vi "mHTprofile.vi"(0 "Gamma0":dbl caption="Gamma0 (0)" format="%#_13g", 1 "Gamma2":dbl caption="Gamma2 (0)" format="%#_13g", 2 "Delta0":dbl caption="Delta0 (0)" format="%#_13g", 3 "Delta2":dbl caption="Delta2 (0)" format="%#_13g", 4 "NuOptRe":dbl caption="NuOptRe (0)" format="%#_13g", 5 "NuOptIm":dbl caption="NuOptIm (0)" format="%#_13g", 6 "Xlm":dbl caption="Xlm (0)" format="%#_13g", 7 "nu0":dbl caption="nu0 (0)" format="%#_13g", 8 "Ylm":dbl caption="Ylm (0)" format="%#_13g", 9 "GammaD":dbl caption="GammaD (0)" format="%#_13g", 10 "alpha":dbl=10.0 caption="alpha (10)" format="%#_13g", 11 "nu":dbl format="%#_13g", 12 "disp":enum32{"Absorption", "Dispersion"}(ring) caption="disp (Absorption)") -> (18 "mHT":dbl=nan format="%#_16g")   [LabVIEW 2015]
panel:
  # "modified Hartman Tran profile"
  # "Subroutine to compute the complex normalized spectral-line shape using mHT model\n\nStandard Input Parameters:\n--------------------\nnu0     : Unperturbed line position in cm-1 (default: 0).\nGammaD  : Doppler broadening in cm-1 (default: 0).\nGamma0  : Speed-averaged line-width in cm-1 (default: 0).       \nGamma2  : Quadratic speed dependence parameter of the line-width in cm-1 (default: 0).\nDelta0  : Speed-averaged line-shift in cm-1 (default: 0).\nDelta2  : Quadratic speed dependence parameter of the line-shift in cm-1 (default: 0).   \nNuOptRe : Real part of the complex Dicke parameter in cm-1 (default: 0).\nNuOptIm : Imaginary part of the complex Dicke parameter in cm-1 (default: 0).    \nnu      : Current WaveNumber in cm-1.\nYlm     : Imaginary part of the 1st order (Rosenkranz) line mixing coefficients, dimensionless (default: 0).\nXlm     : Real part of the 1st order (Rosenkranz) line mixing coefficients, dimensionless (default: 0).\nalpha   : Mass ratio in the molecule for calculating beta-correction, applicable up to alpha=5, \n          dimensionless (default: 10).\ndisp    : Boolean trigger for including dispersion profile in the output (default: Absorption).\n\nThe function has one outputs:\n--------------------\n(1)     : Real or imaginary (depending on disp value) part of the normalized spectral shape in cm."
  # "Input Section"
  # "Output Section"
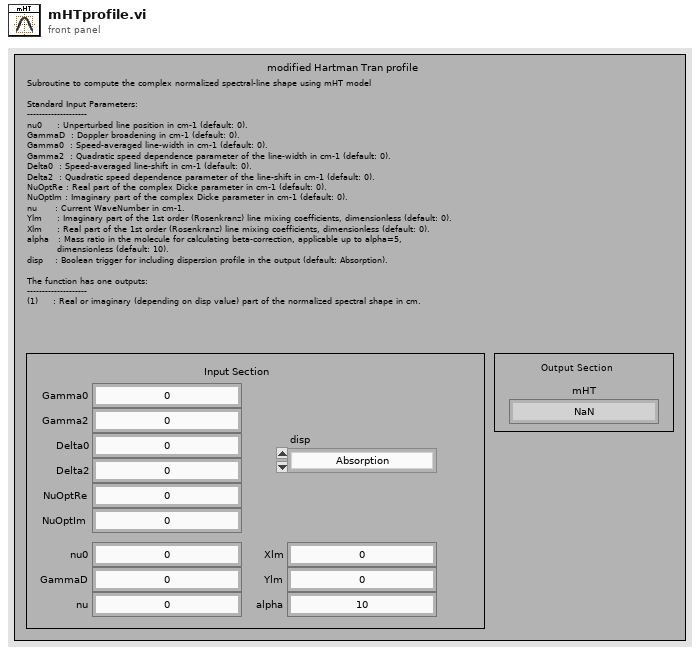
[diagram p1: front panel]
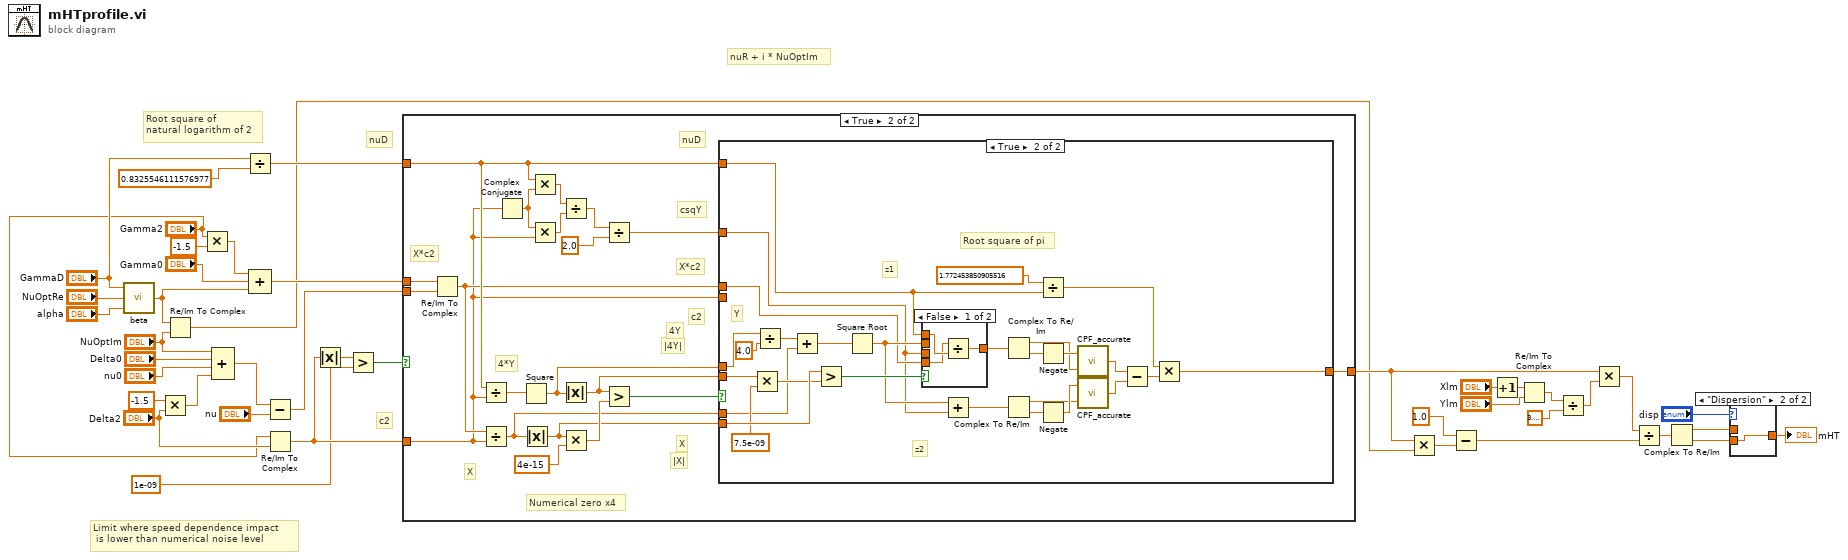
[diagram p0: block diagram]
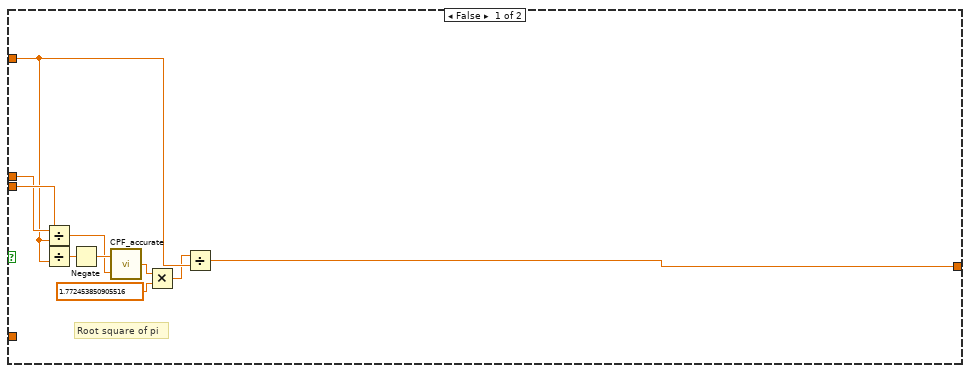
[diagram p3: hidden frame]
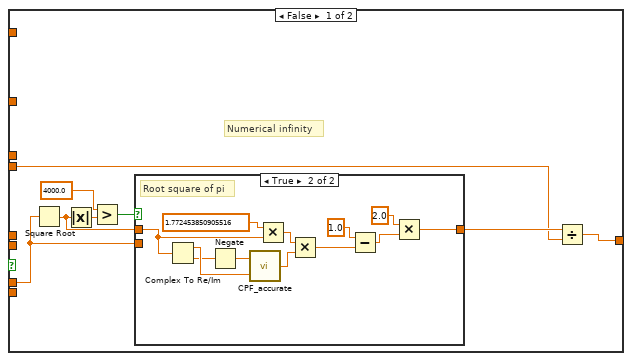
[diagram p4: hidden frame]
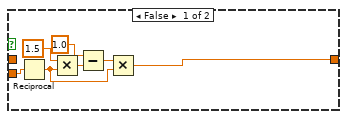
[diagram p5: hidden frame]
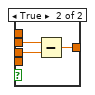
[diagram p6: hidden frame]
diagram:
  # "nuR + i * NuOptIm"
  # "nuD"
  # "c2"
  # "Limit where speed dependence impact\n is lower than numerical noise level"
  # "Root square of\nnatural logarithm of 2"
  n1 = call "beta.vi"("alpha"="alpha", "NuOptRe"="NuOptRe", "GammaD"="GammaD") -> ("nuR"=w11:dbl)
  n2 = Multiply(x=-1.5 ("y"), y="Delta2") -> (x*y=w3:dbl)
  n3 = Re/Im To Complex(1:"NuOptIm", 2:w11) -> (0:w25:cdb)
  n4 = Multiply(x="Gamma2", y=-1.5) -> (x*y=w10:dbl)
  n5 = Compound Arithmetic op=ADD("NuOptIm", "Delta0", "nu0", w3) -> (w2:dbl)
  n6 = Divide(x="GammaD", y=0.8325546111576977 ("sln2")) -> (x/y=w32:dbl)
  n7 = Compound Arithmetic op=ADD(w10, "Gamma0", w11) -> (w34:dbl)
  n8 = Subtract(x=w2, y="nu") -> (x-y=w33:dbl)
  n9 = Re/Im To Complex(1:"Delta2", 2:"Gamma2") -> (0:w6:cdb)
  n10 = Absolute Value(x=w6) -> (abs(x)=w36:dbl)
  n11 = Greater?(x=w36, y=1e-09) -> (0:w35:bool)
  n12 = case shown="True" w35 {
    tunnel: w34 -> [w50 w71]
    tunnel: w33 -> [w51 w55]
    tunnel: w32 -> [w44 w56]
    tunnel: w6 -> [_ w53]
    tunnel: [w42 w57] -> w26
    frame False {
      # "Root square of pi"
      n13 = Divide(x=w50, y=w44) -> (x/y=w47:dbl)
      n14 = Divide(x=w51, y=w44) -> (x/y=w49:dbl)
      n15 = Negate(x=w49) -> (-x=w48:dbl)
      n16 = call "CPF_accurate.vi"("y"=w47, "x"=w48) -> ("CPF Value"=w46:cdb)
      n17 = Multiply(x=w46, y=1.772453850905516) -> (x*y=w43:cdb)
      n18 = Divide(x=w43, y=w44) -> (x/y=w42:cdb)
    }
    frame True {
      # "|4Y|"
      # "4Y"
      # "|X|"
      # "X"
      # "4*Y"
      # "X"
      # "c2"
      # "X*c2"
      # "csqY"
      # "nuD"
      # "X*c2"
      # "Numerical zero x4"
      n19 = Re/Im To Complex(1:w55, 2:w71) -> (0:w54:cdb)
      n20 = Divide(x=w56, y=w53) -> (x/y=w70:cdb)
      n21 = Divide(x=w54, y=w53) -> (x/y=w61:cdb)
      n22 = Complex Conjugate(1:w53) -> (0:w67:cdb)
      n23 = Square(x=w70) -> (x^2=w60:cdb)
      n24 = Absolute Value(x=w61) -> (abs(x)=w59:dbl)
      n25 = Multiply(x=w56, y=w67) -> (x*y=w66:cdb)
      n26 = Multiply(x=w67, y=w53) -> (x*y=w65:cdb)
      n27 = Divide(x=w66, y=w65) -> (x/y=w64:cdb)
      n28 = Absolute Value(x=w60) -> (abs(x)=w58:dbl)
      n29 = Multiply(x=w59, y=4e-15 ("sln2")) -> (x*y=w69:dbl)
      n30 = Divide(x=w64, y=2.0) -> (x/y=w62:cdb)
      n31 = Greater?(x=w58, y=w69) -> (0:w68:bool)
      n32 = case shown="True" w68 {
        tunnel: w62 -> [_ w100]
        tunnel: w61 -> [w76 w114]
        tunnel: w53 -> [w78 _]
        tunnel: w60 -> [_ w123]
        tunnel: w59 -> [_ w118]
        tunnel: w58 -> [_ w117]
        tunnel: w54 -> [_ w101]
        tunnel: w56 -> [_ w99]
        tunnel: [w72 w102] -> w57
        frame False {
          # "Numerical infinity"
          n33 = Square Root(x=w76) -> (sqrt(x)=w73:cdb)
          n34 = Absolute Value(x=w73) -> (abs(x)=w77:dbl)
          n35 = Greater?(x=4000.0 ("sln2"), y=w77) -> (0:w74:bool)
          n36 = case shown="True" w74 {
            tunnel: w76 -> [w86 _]
            tunnel: w73 -> [_ w87]
            tunnel: [w81 w88] -> w79
            frame False {
              n37 = Reciprocal(x=w86) -> (1/x=w80:cdb)
              n38 = Multiply(x=1.5, y=w80) -> (x*y=w84:cdb)
              n39 = Subtract(x=1.0, y=w84) -> (x-y=w82:cdb)
              n40 = Multiply(x=w82, y=w80) -> (x*y=w81:cdb)
            }
            frame True {
              # "Root square of pi"
              n41 = Complex To Re/Im(x + iy=w87) -> (x=w97:dbl, y=w96:dbl)
              n42 = Negate(x=w96) -> (-x=w98:dbl)
              n43 = call "CPF_accurate.vi"("y"=w97, "x"=w98) -> ("CPF Value"=w94:cdb)
              n44 = Multiply(x=1.772453850905516, y=w87) -> (x*y=w93:cdb)
              n45 = Multiply(x=w93, y=w94) -> (x*y=w92:cdb)
              n46 = Subtract(x=1.0, y=w92) -> (x-y=w90:cdb)
              n47 = Multiply(x=2.0, y=w90) -> (x*y=w88:cdb)
            }
          }
          n48 = Divide(x=w79, y=w78) -> (x/y=w72:cdb)
        }
        frame True {
          # "z2"
          # "z1"
          # "Y"
          # "Root square of pi"
          n49 = Multiply(x=w117, y=7.5e-09) -> (x*y=w115:dbl)
          n50 = Divide(x=w123, y=4.0) -> (x/y=w125:cdb)
          n51 = Add(x=w125, y=w114) -> (x+y=w126:cdb)
          n52 = Greater?(x=w118, y=w115) -> (0:w122:bool)
          n53 = Square Root(x=w126) -> (sqrt(x)=w120:cdb)
          n54 = case shown="False" w122 {
            tunnel: w120 -> [_ w132]
            tunnel: w100 -> [_ w131]
            tunnel: [w128 w130] -> w121
            tunnel: w99 -> [w129 _]
            tunnel: w101 -> [w127 _]
            frame False {
              n55 = Divide(x=w127, y=w129) -> (x/y=w128:cdb)
            }
            frame True {
              n56 = Subtract(x=w132, y=w131) -> (x-y=w130:cdb)
            }
          }
          n57 = Add(x=w120, y=w100) -> (x+y=w119:cdb)
          n58 = Complex To Re/Im(x + iy=w121) -> (x=w108:dbl, y=w111:dbl)
          n59 = Complex To Re/Im(x + iy=w119) -> (x=w109:dbl, y=w110:dbl)
          n60 = Divide(x=1.772453850905516, y=w99) -> (x/y=w103:dbl)
          n61 = Negate(x=w111) -> (-x=w113:dbl)
          n62 = Negate(x=w110) -> (-x=w112:dbl)
          n63 = call "CPF_accurate.vi"("y"=w108, "x"=w113) -> ("CPF Value"=w107:cdb)
          n64 = call "CPF_accurate.vi"("y"=w109, "x"=w112) -> ("CPF Value"=w106:cdb)
          n65 = Subtract(x=w107, y=w106) -> (x-y=w104:cdb)
          n66 = Multiply(x=w103, y=w104) -> (x*y=w102:cdb)
        }
      }
    }
  }
  n67 = Multiply(x=w26, y=w25) -> (x*y=w23:cdb)
  n68 = Subtract(x=1.0, y=w23) -> (x-y=w21:cdb)
  n69 = Increment(x="Xlm") -> (x+1=w30:dbl)
  n70 = Re/Im To Complex(1:"Ylm", 2:w30) -> (0:w28:cdb)
  n71 = Divide(x=w28, y=3.141592653589793) -> (x/y=w27:cdb)
  n72 = Multiply(x=w26, y=w27) -> (x*y=w22:cdb)
  n73 = Divide(x=w22, y=w21) -> (x/y=w20:cdb)
  n74 = Complex To Re/Im(x + iy=w20) -> (x=w18:dbl, y=w17:dbl)
  n75 = case shown="\"Dispersion\"" "disp" {
    tunnel: w18 -> [w133 _]
    tunnel: w17 -> [_ w134]
    tunnel: [w133 w134] -> w16
    frame "Absorption", Default {
    }
    frame "Dispersion" {
    }
  }
  "mHT" <- w16
